vi "MY_NEW_STRUCTURE.vi"(8 "Dataflow In":errorcluster) -> (0 "Dataflow Out":errorcluster)   [LabVIEW 2019]
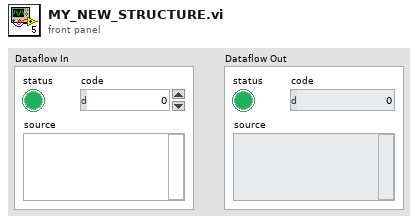
[diagram p1: front panel]
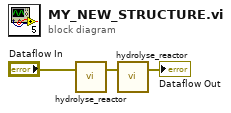
[diagram p0: block diagram]
diagram:
  n1 = call "hydrolyse_reactor.vi"("Dataflow In"="Dataflow In") -> ("Dataflow Out"=w2:errorcluster)  [unwired: 2 in]
  n2 = call "hydrolyse_reactor.vi"("Dataflow In"=w2) -> ("Dataflow Out"=→"Dataflow Out":errorcluster)  [unwired: 2 in]
